vi "Init_DAC_MCP4728.vi"(8 "error in (no error)":errorcluster, 10 "LINX Resource in":T1, 11 "I2C Channel (0)":u8) -> (0 "error out":errorcluster, 3 "LINX Resource out":T1)   [LabVIEW 2018]
uses:
  <vilib>/MakerHub/LINX/Private/Type Defs/LINX Ref.ctl
  <vilib>/MakerHub/LINX/Private/Type Defs/Platform.ctl
  <vilib>/MakerHub/LINX/Private/Type Defs/Interface.ctl
  <vilib>/MakerHub/LINX/Private/Device/Type Defs/LINX Device Config.ctl
  <vilib>/MakerHub/LINX/Private/Device/Type Defs/TCP Config.ctl
  <vilib>/MakerHub/LINX/Private/Device/Type Defs/Channels.ctl
  <vilib>/MakerHub/LINX/Private/Local IO/LinxI2cWrite.vi
  <vilib>/MakerHub/LINX/Public/Utilities/Check Channel.vi
  <vilib>/MakerHub/LINX/Private/Utilties/Generate Error.vi
  <vilib>/MakerHub/LINX/LMH-LINX.lvlib
  <vilib>/MakerHub/LINX/Private/Device/Device.lvlib
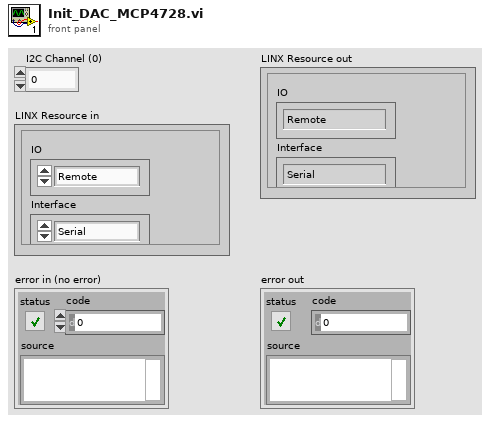
[diagram p1: front panel]
types:
  T1 = typedef "LMH-LINX.lvlib/LINX Ref.ctl" = cluster{"IO":T2, "Interface":T3, "LINX Device Config":T4}
  T2 = typedef "LMH-LINX.lvlib/Platform.ctl" = enum16{"Remote", "Local"}
  T3 = typedef "LMH-LINX.lvlib/Interface.ctl" = enum16{"Serial", "TCP"}
  T4 = typedef "LMH-LINX.lvlib/Device.lvlib/LINX Device Config.ctl" = cluster{"Interface":T3, "COM Port":refnum<visa-resource-name>, "TCP Configuration":T5, "Device Family":u8, "Device ID":u8, "Device Name":string, "TCP Ref":refnum<k5>, "Channels":T6}
  T5 = typedef "LMH-LINX.lvlib/Device.lvlib/TCP Config.ctl" = cluster{"IP Address":string, "Port":u16}
  T6 = typedef "LMH-LINX.lvlib/Channels.ctl" = cluster{"DI":u8[], "DO":u8[], "AI":u8[], "AO":u8[], "PWM":u8[], "QE":u8[], "UART":u8[], "I2C 2":u8[], "SPI":u8[], "CAN":u8[], "Servo":u8[], "AI Ref (V)":dbl, "AI Resolution (Bits)":u8, "AO Ref (V)":dbl, "AO Resolution (Bits)":u8}
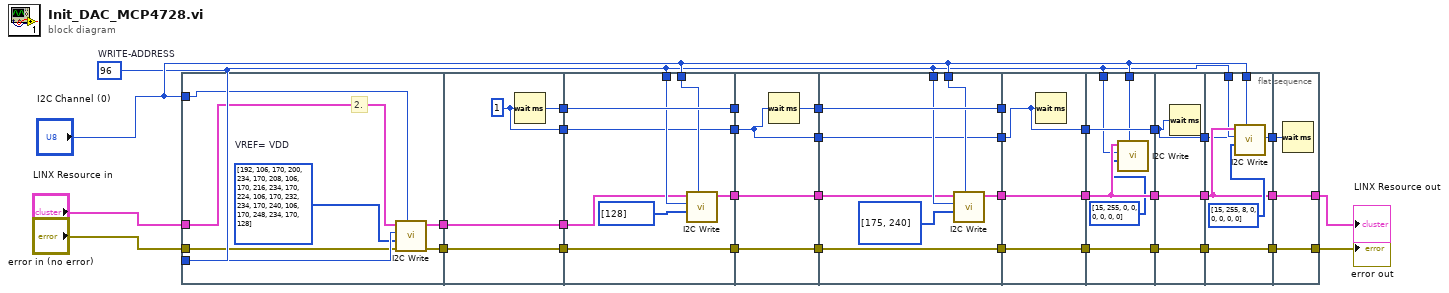
[diagram p0: block diagram]
diagram:
  w3 = u8 96  # WRITE-ADDRESS
  n1 = flat-sequence {
    tunnel: "LINX Resource in" -> [w43]
    tunnel: w3 -> [w41]
    tunnel: "error in (no error)" -> [w40]
    tunnel: "I2C Channel (0)" -> [w38]
    tunnel: [w42] -> w36
    tunnel: [w39] -> w35
    tunnel: w36 -> [w47]
    tunnel: w35 -> [w46]
    tunnel: [w47] -> w34
    tunnel: [w46] -> w33
    tunnel: [w45] -> w32
    tunnel: [w44] -> w31
    tunnel: w34 -> [w50]
    tunnel: w33 -> [w55]
    tunnel: [w49] -> w30
    tunnel: [w55] -> w29
    tunnel: w32 -> [w54]
    tunnel: [w54] -> w28
    tunnel: "I2C Channel (0)" -> [w53]
    tunnel: w3 -> [w52]
    tunnel: w31 -> [w48]
    tunnel: [w48] -> w27
    tunnel: w30 -> [w59]
    tunnel: w29 -> [w58]
    tunnel: [w59] -> w26
    tunnel: [w58] -> w25
    tunnel: w28 -> [_]
    tunnel: [w57] -> w24
    tunnel: w27 -> [w56]
    tunnel: [w56] -> w23
    tunnel: w26 -> [w62]
    tunnel: w25 -> [w67]
    tunnel: [w61] -> w22
    tunnel: [w67] -> w21
    tunnel: w24 -> [w66]
    tunnel: [w66] -> w20
    tunnel: "I2C Channel (0)" -> [w65]
    tunnel: w3 -> [w64]
    tunnel: w23 -> [w60]
    tunnel: [w60] -> w19
    tunnel: w22 -> [w70]
    tunnel: w21 -> [w69]
    tunnel: w20 -> [_]
    tunnel: w19 -> [w68]
    tunnel: [w70] -> w18
    tunnel: [w69] -> w17
    tunnel: [w68] -> w16
    tunnel: w18 -> [w74]
    tunnel: w17 -> [w76]
    tunnel: [w74] -> w15
    tunnel: [w76] -> w14
    tunnel: w16 -> [w75]
    tunnel: [w75] -> w13
    tunnel: "I2C Channel (0)" -> [w72]
    tunnel: w3 -> [w71]
    tunnel: w15 -> [w79]
    tunnel: w14 -> [w78]
    tunnel: w13 -> [w77]
    tunnel: [w79] -> w12
    tunnel: [w78] -> w11
    tunnel: [w77] -> w10
    tunnel: w12 -> [w83]
    tunnel: w11 -> [w85]
    tunnel: [w83] -> w9
    tunnel: [w85] -> w8
    tunnel: "I2C Channel (0)" -> [w82]
    tunnel: w3 -> [w81]
    tunnel: w10 -> [w80]
    tunnel: [w80] -> w7
    tunnel: [w87] -> w5
    tunnel: [w88] -> w6
    tunnel: w9 -> [w88]
    tunnel: w8 -> [w87]
    tunnel: w7 -> [w86]
    frame #0 {
      w37 = u8[] [192, 106, 170, 200, 234, 170, 208, 106, 170, 216, 234, 170, 224, 106, 170, 232, 234, 170, 240, 106, 170, 248, 234, 170, 128]  # VREF= VDD
      # "2."
      n2 = call <vilib>:"I2C Write.vi"("I2C Channel"=w38, "Error In"=w40, "Data"=w37, "I2C Slave Address (0)"=w41, "LINX Resource"=w43) -> ("Error Out"=w39:errorcluster, "LINX Resource"=w42:T1)  [unwired: 5 in]
    }
    frame #1 {
      w44 = u32 1 ("milliseconds to wait")
      n3 = Wait (ms)(milliseconds to wait=w44) -> (millisecond timer value=w45:u32)
    }
    frame #2 {
      n4 = call <vilib>:"I2C Write.vi"("I2C Channel"=w53, "Data"=u8[] [128], "I2C Slave Address (0)"=w52, "LINX Resource"=w50) -> ("LINX Resource"=w49:T1)  [unwired: 6 in, 1 out]
    }
    frame #3 {
      n5 = Wait (ms)(milliseconds to wait=w56) -> (millisecond timer value=w57:u32)
    }
    frame #4 {
      n6 = call <vilib>:"I2C Write.vi"("I2C Channel"=w65, "Data"=u8[] [175, 240], "I2C Slave Address (0)"=w64, "LINX Resource"=w62) -> ("LINX Resource"=w61:T1)  [unwired: 6 in, 1 out]
    }
    frame #5 {
      n7 = Wait (ms)(milliseconds to wait=w68) -> ()  [unwired: 1 out]
    }
    frame #6 {
      n8 = call <vilib>:"I2C Write.vi"("I2C Channel"=w72, "Data"=u8[] [15, 255, 0, 0, 0, 0, 0, 0] ("X"), "I2C Slave Address (0)"=w71, "LINX Resource"=w74) -> ()  [unwired: 6 in, 2 out]
    }
    frame #7 {
      n9 = Wait (ms)(milliseconds to wait=w77) -> ()  [unwired: 1 out]
    }
    frame #8 {
      n10 = call <vilib>:"I2C Write.vi"("I2C Channel"=w82, "Data"=u8[] [15, 255, 8, 0, 0, 0, 0, 0] ("number"), "I2C Slave Address (0)"=w81, "LINX Resource"=w83) -> ()  [unwired: 6 in, 2 out]
    }
    frame #9 {
      n11 = Wait (ms)(milliseconds to wait=w86) -> ()  [unwired: 1 out]
    }
  }
  "LINX Resource out" <- w6
  "error out" <- w5
